vi "Get Data.vi"(8 "error in":errorcluster, 11 "Temperature Device in":refnum<class "Temperature Device.lvclass">) -> (0 "error out":errorcluster, 2 "Data":dbl[](array[numeric]), 3 "Temperature Device out":refnum<class "Temperature Device.lvclass">)   [LabVIEW 2015, in "Temperature Device.lvclass"]
uses:
  Temperature Device.lvclass
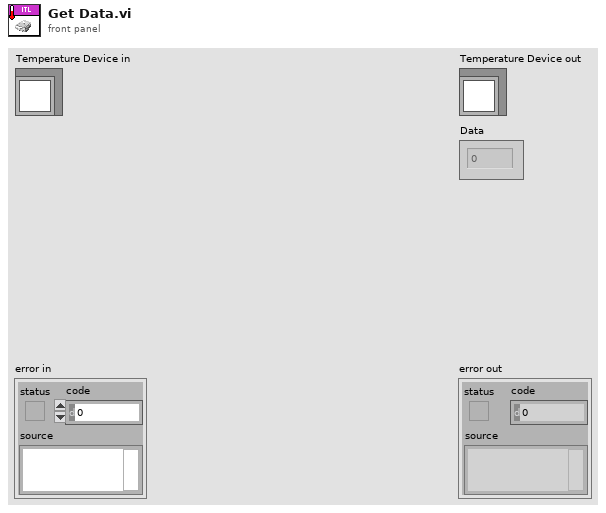
[diagram p1: front panel]
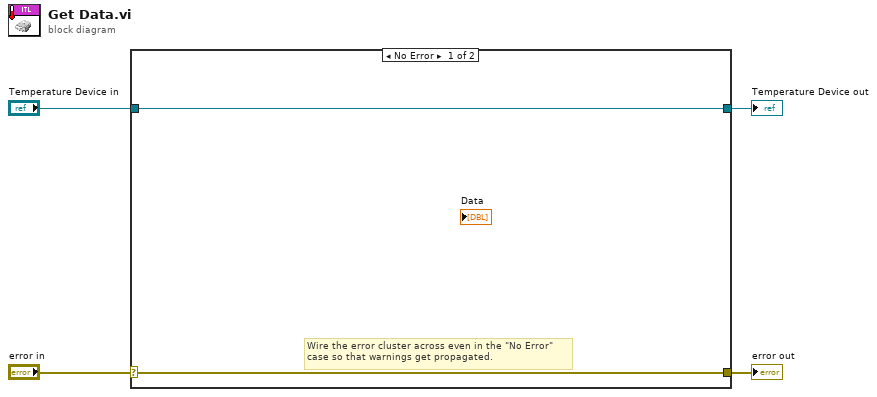
[diagram p0: block diagram]
diagram:
  n1 = case shown="No Error" "error in" {
    selector: "error in" -> [w5 w8]
    tunnel: [w5 w8] -> w3
    tunnel: [w6 w7] -> w1
    tunnel: "Temperature Device in" -> [w6 w7]
    frame No Error {
      # "Wire the error cluster across even in the \"No Error\"\ncase so that warnings get propagated."
    }
    frame Error {
    }
  }
  "error out" <- w3
  "Temperature Device out" <- w1
